vi "DangerEnemy.vi"(10 "IA Input":T1={"our_robots"=[], "enemy_robots"=[], "balls"=[], "geometry"={"line_width"=0, "field_length"=0, "field_width"=0, "boundary_width"=0, "referee_width"=0, "goal_width"=0, "goal_depth"=0, "goal_wall_width"=0, "center_circle_radius"=0, "defense_radius"=0, "defense_stretch"=0, "free_kick_from_defense_dist"=0, "penalty_spot_from_field_line_dist"=0, "penalty_line_from_spot_dist"=0}, "IA Judge"={"stage"="", "command"="", "our_goalie_id"=0.0, "enemy_goalie_id"=0.0, "command enum"=enum."Halt", "Time"=enum."Azul"}, "Received Timestamp"=timestamp(0 s since 1904-01-01), "Events"={"Touch"=FALSE, "Ball out"=FALSE, "id touch"=0.0, "Ball out of \nVision"=FALSE, "Ball inside \nGoalie area"=FALSE, "Robot not responding"=FALSE, "Robots responding status"=[1.0, 1.0, 1.0, 1.0, 1.0, 1.0], "Enemy Ball \nPossession"=FALSE, "Pass State"=FALSE, "id end of pass"=0.0, "Kick"=FALSE, "Id ini Possession"=0.0, "Ball Possesion"=FALSE, "Id Possesion"=0.0}}) -> (0 "Pos do segundo inimigo\nperigoso":dbl[](array[numeric]), 1 "id do segundo inimigo\nmais perigoso":u32, 2 "Pos do inimigo\nperigoso":dbl[](array[numeric]), 3 "id do inimigo\nmais perigoso":u32)   [LabVIEW 2017]
uses:
  Core/AI Input.ctl
  Core/AI Robot.ctl
  Functions Enum.ctl
  AttackerStates.ctl
  Path Planning/RRT/PathDests.ctl
  Path Planning/RRT/PathDest.ctl
  Core/AI Ball.ctl
  Core/Field Size.ctl
  Core/AI Judge.ctl
  Command Enum.ctl
  Util/Events/Events.ctl
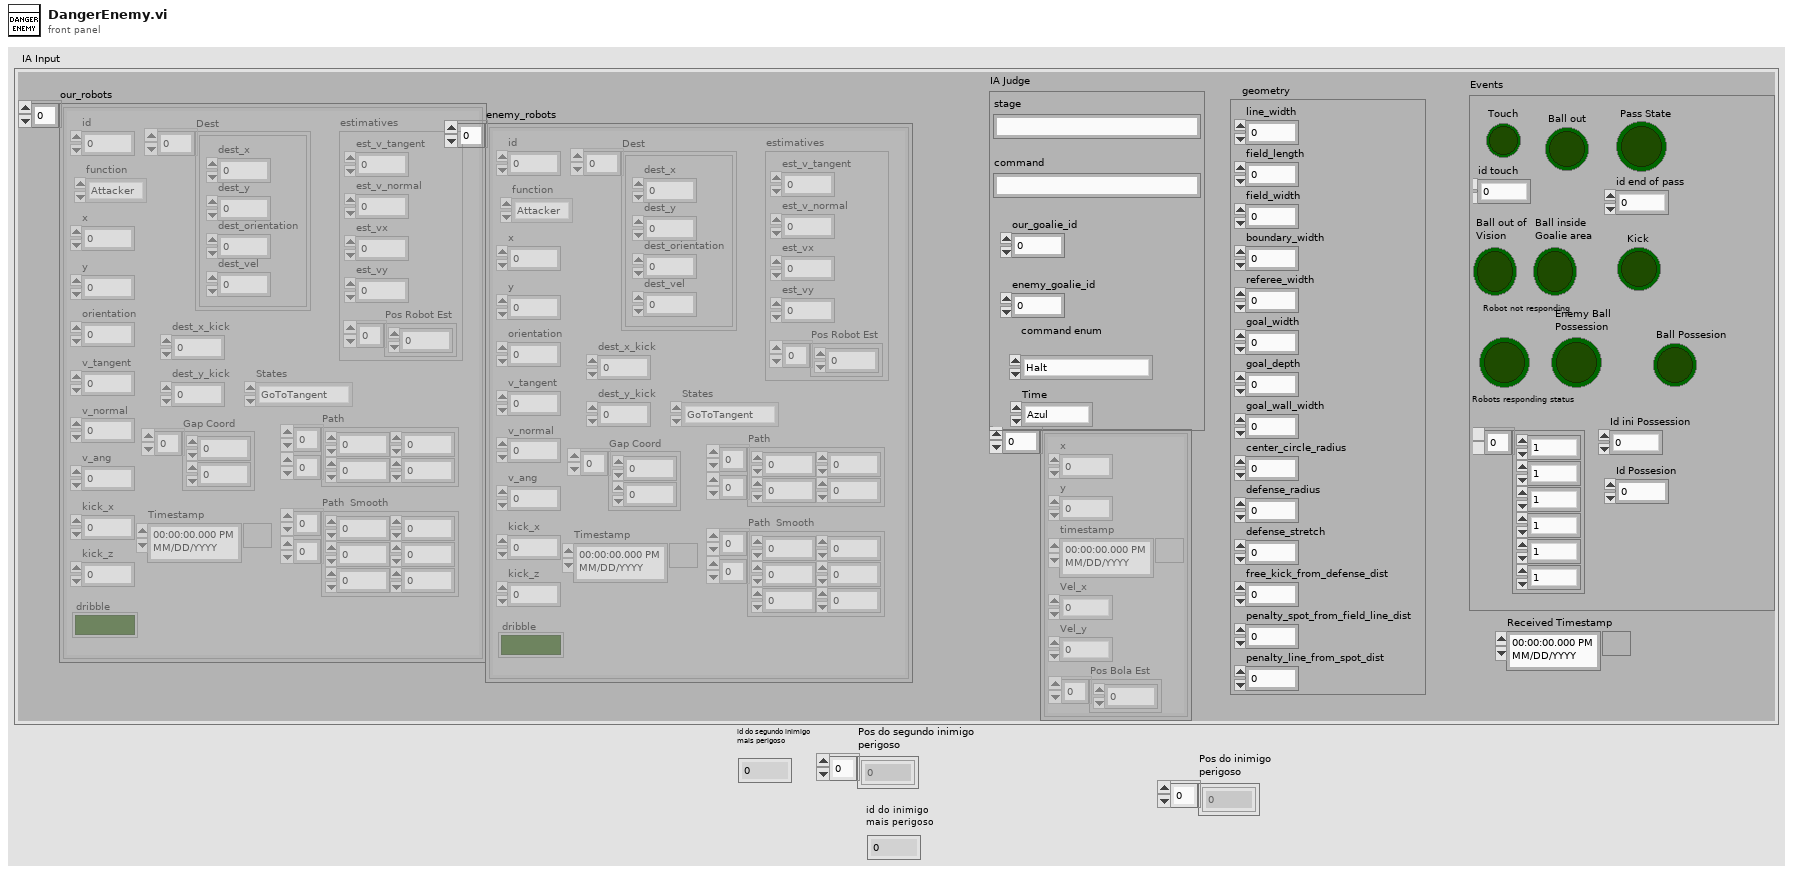
[diagram p1: front panel]
types:
  T1 = typedef "AI Input.ctl" = cluster{"our_robots":T2[], "enemy_robots":T2[], "balls":T7[], "geometry":T8, "IA Judge":T9, "Received Timestamp":timestamp, "Events":T11}
  T2 = typedef "AI Robot.ctl" = cluster{"id":u32, "function":T3, "x":dbl, "y":dbl, "orientation":dbl, "v_tangent":dbl, "v_normal":dbl, "v_ang":dbl, "kick_x":dbl, "kick_z":dbl, "dribble":bool, "Timestamp":timestamp, "estimatives":cluster{"est_v_tangent":dbl, "est_v_normal":dbl, "est_vx":dbl, "est_vy":dbl, "Pos Robot Est":dbl[]}, "dest_x_kick":dbl, "dest_y_kick":dbl, "Gap Coord":dbl[], "States":T4, "Path ":dbl[][], "Path  Smooth":dbl[][], "Dest":T5}
  T3 = typedef "Functions Enum.ctl" = enum16{"Attacker", "Goalie", "Defender", "Striker", "Goto 0", "Dummy", "Kicker", "ZigZag"}
  T4 = typedef "AttackerStates.ctl" = enum16{"Pass", "GoToTangent", "BallGetting", "GoToKick", ""}
  T5 = typedef "PathDests.ctl" = T6[]
  T6 = typedef "PathDest.ctl" = cluster{"dest_x":dbl, "dest_y":dbl, "dest_orientation":dbl, "dest_vel":dbl}
  T7 = typedef "AI Ball.ctl" = cluster{"x":dbl, "y":dbl, "timestamp":timestamp, "Vel_x":dbl, "Vel_y":dbl, "Pos Bola Est":dbl[]}
  T8 = typedef "Field Size.ctl" = cluster{"line_width":u32, "field_length":u32, "field_width":u32, "boundary_width":u32, "referee_width":u32, "goal_width":u32, "goal_depth":u32, "goal_wall_width":u32, "center_circle_radius":u32, "defense_radius":u32, "defense_stretch":u32, "free_kick_from_defense_dist":u32, "penalty_spot_from_field_line_dist":u32, "penalty_line_from_spot_dist":u32}
  T9 = typedef "AI Judge.ctl" = cluster{"stage":string, "command":string, "our_goalie_id":dbl, "enemy_goalie_id":dbl, "command enum":T10, "Time":enum16{"Azul", "Amarelo"}}
  T10 = typedef "Command Enum.ctl" = enum16{"Halt", "Stop", "Force Start", "PKA Normal Start", "Prepare Kickoff Ally", "PKE Normal Start", "Prepare Kickoff Enemy", "Prepare Penalty Ally", "PPA Normal Start", "Prepare Penalty Enemy", "PPE Normal Start", "Direct Free Enemy", "Direct Free Ally", "Indirect Free Enemy", "Indirect Free Ally", "Timeout Enemy", "Timeout Ally", "Goal Enemy", "Goal Ally", "Ball Placement Enemy", "Ball Placement Ally", "Normal Half Time", "Extra Time Break", "Extra Half Time", "None", "Post Game"}
  T11 = typedef "Events.ctl" = cluster{"Touch":bool, "Ball out":bool, "id touch":dbl, "Ball out of \nVision":bool, "Ball inside \nGoalie area":bool, "Robot not responding":bool, "Robots responding status":dbl[], "Enemy Ball \nPossession":bool, "Pass State":bool, "id end of pass":dbl, "Kick":bool, "Id ini Possession":dbl, "Ball Possesion":bool, "Id Possesion":dbl}
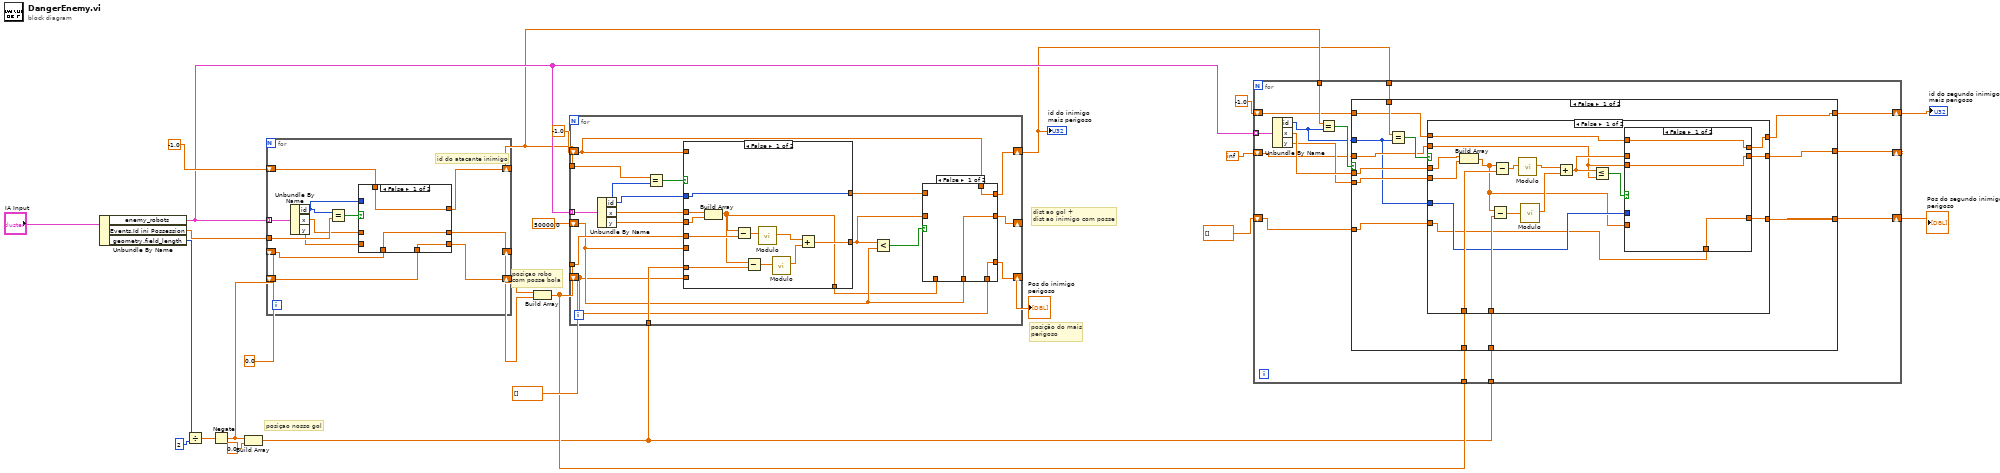
[diagram p0: block diagram]
diagram:
  # "dist ao gol +\ndist ao inimigo com posse"
  # "posição do mais\nperigoso"
  # "posiçao nosso gol"
  # "posiçao robo\ncom posse bola"
  n1 = Unbundle By Name("IA Input") -> ("enemy_robots"=w10:T2[], "Events.Id ini Possession"=w24:dbl, "geometry.field_length"=w21:u32)
  n2 = Divide(x=w21, y=u32 2) -> (x/y=w19:dbl)
  n3 = Negate(x=w19) -> (-x=w11:dbl)
  n4 = Build Array(w11, 0.0 ("element")) -> (w2:dbl[])
  n5 = for {
    tunnel: w10 -> [w37] mode=indexing
    tunnel: w24 -> [w36]
    shift-right: [w31] -> w9
    shift-left: -1.0 ("id") -> [w28]
    shift-right: [w30] -> w23
    shift-left: w11 -> [w27]
    shift-right: [w29] -> w22
    shift-left: 0.0 ("y") -> [w26]
    # "id do atacante inimigo"
    n6 = Unbundle By Name(w37) -> ("id"=w34:u32, "x"=w33:dbl, "y"=w32:dbl)
    n7 = Equal?(x=w34, y=w36) -> (x = y?=w35:bool)
    n8 = case shown="False" w35 {
      tunnel: w34 -> [_ w43]
      tunnel: w33 -> [_ w42]
      tunnel: w32 -> [_ w41]
      tunnel: [w40 w43] -> w31
      tunnel: [w39 w42] -> w30
      tunnel: [w38 w41] -> w29
      tunnel: w28 -> [w40 _]
      tunnel: w27 -> [w39 _]
      tunnel: w26 -> [w38 _]
      frame False {
      }
      frame True {
      }
    }
  }
  n9 = Build Array(w23, w22) -> (w3:dbl[])
  n10 = for {
    tunnel: w10 -> [w61] mode=indexing
    tunnel: w9 -> [w60]
    tunnel: w3 -> [w56]
    tunnel: w2 -> [w55]
    shift-right: [w52] -> _
    shift-left: 50000.0 -> [w51]
    shift-right: [w48] -> w4
    shift-left: -1.0 ("id") -> [w45]
    shift-right: [w46] -> w16
    shift-left: dbl[] [] -> [w44]
    n11 = Unbundle By Name(w61) -> ("id"=w50:u32, "x"=w58:dbl, "y"=w57:dbl)
    n12 = Equal?(x=w60, y=w50) -> (x = y?=w59:bool)
    n13 = case shown="False" w59 {
      tunnel: w58 -> [w78 _]
      tunnel: w57 -> [w77 _]
      tunnel: w56 -> [w76 _]
      tunnel: w55 -> [w74 _]
      tunnel: [w70 w81] -> w53
      tunnel: w51 -> [_ w81]
      tunnel: w50 -> [w69 _]
      tunnel: [w69 w80] -> w49
      tunnel: [w68 w79] -> w47
      tunnel: w45 -> [_ w80]
      tunnel: w44 -> [_ w79]
      frame False {
        n14 = Build Array(w78, w77) -> (w68:dbl[])
        n15 = Subtract(x=w68, y=w76) -> (x-y=w75:dbl[])
        n16 = Subtract(x=w68, y=w74) -> (x-y=w73:dbl[])
        n17 = call "Modulo.vi"("2D vector"=w75) -> ("Modulo"=w72:dbl)  [unwired: 10 in]
        n18 = call "Modulo.vi"("2D vector"=w73) -> ("Modulo"=w71:dbl)  [unwired: 10 in]
        n19 = Add(x=w72, y=w71) -> (x+y=w70:dbl)
      }
      frame True {
      }
    }
    n20 = Less?(x=w53, y=w51) -> (x < y?=w54:bool)
    n21 = case shown="False" w54 {
      tunnel: w53 -> [_ w67]
      tunnel: [w64 w67] -> w52
      tunnel: w51 -> [w64 _]
      tunnel: [w63 w66] -> w48
      tunnel: w49 -> [_ w66]
      tunnel: w45 -> [w63 _]
      tunnel: w47 -> [_ w65]
      tunnel: [w62 w65] -> w46
      tunnel: w44 -> [w62 _]
      frame False {
      }
      frame True {
      }
    }
  }
  "id do inimigo\nmais perigoso" <- w4
  "Pos do inimigo\nperigoso" <- w16
  n22 = for {
    tunnel: w10 -> [w96] mode=indexing
    tunnel: w9 -> [w95]
    shift-right: [w93] -> w1
    shift-left: -1.0 -> [w92]
    shift-right: [w91] -> _
    shift-left: inf -> [w82]
    shift-right: [w90] -> w5
    shift-left: dbl[] [] -> [w89]
    tunnel: w4 -> [w87]
    tunnel: w3 -> [w84]
    tunnel: w2 -> [w83]
    n23 = Unbundle By Name(w96) -> ("id"=w88:u32, "x"=w86:dbl, "y"=w85:dbl)
    n24 = Equal?(x=w95, y=w88) -> (x = y?=w94:bool)
    n25 = case shown="False" w94 {
      tunnel: w92 -> [w107 w139]
      tunnel: [w106 w139] -> w93
      tunnel: w82 -> [w105 w138]
      tunnel: [w104 w138] -> w91
      tunnel: w89 -> [w103 w137]
      tunnel: [w102 w137] -> w90
      tunnel: w88 -> [w97 _]
      tunnel: w87 -> [w109 _]
      tunnel: w86 -> [w101 _]
      tunnel: w85 -> [w100 _]
      tunnel: w84 -> [w99 _]
      tunnel: w83 -> [w98 _]
      frame False {
        n26 = Equal?(x=w109, y=w97) -> (x = y?=w108:bool)
        n27 = case shown="False" w108 {
          tunnel: [w118 w136] -> w106
          tunnel: w107 -> [w116 w136]
          tunnel: w105 -> [w110 w135]
          tunnel: [w114 w135] -> w104
          tunnel: w103 -> [w111 w134]
          tunnel: [w112 w134] -> w102
          tunnel: w101 -> [w127 _]
          tunnel: w100 -> [w126 _]
          tunnel: w99 -> [w125 _]
          tunnel: w98 -> [w122 _]
          tunnel: w97 -> [w117 _]
          frame False {
            n28 = Build Array(w127, w126) -> (w113:dbl[])
            n29 = Subtract(x=w113, y=w122) -> (x-y=w121:dbl[])
            n30 = Subtract(x=w113, y=w125) -> (x-y=w124:dbl[])
            n31 = call "Modulo.vi"("2D vector"=w124) -> ("Modulo"=w123:dbl)  [unwired: 10 in]
            n32 = call "Modulo.vi"("2D vector"=w121) -> ("Modulo"=w120:dbl)  [unwired: 10 in]
            n33 = Add(x=w123, y=w120) -> (x+y=w115:dbl)
            n34 = Less Or Equal?(x=w115, y=w110) -> (x <= y?=w119:bool)
            n35 = case shown="False" w119 {
              tunnel: [w130 w133] -> w118
              tunnel: w117 -> [_ w133]
              tunnel: w116 -> [w130 _]
              tunnel: [w128 w132] -> w114
              tunnel: w115 -> [_ w132]
              tunnel: [w129 w131] -> w112
              tunnel: w113 -> [_ w131]
              tunnel: w111 -> [w129 _]
              tunnel: w110 -> [w128 _]
              frame False {
              }
              frame True {
              }
            }
          }
          frame True {
          }
        }
      }
      frame True {
      }
    }
  }
  "id do segundo inimigo\nmais perigoso" <- w1
  "Pos do segundo inimigo\nperigoso" <- w5
